vi "Lab2_FM.vi"() -> ()   [LabVIEW 2019]
uses:
  <vilib>/express/express analysis/Spectral/Block/exnSpectralBlock spectral measurements RMS poly.vi
  <vilib>/express/express analysis/Spectral/Block/exnSpectralBlock spectral measurements RMS DDT.vi
  <vilib>/express/express analysis/Spectral/XNode/ExpressSpectralMeasurementsBlockNode.xnode
panel:
  in  "stop":bool
  out "Time Domain":dynamicdata(graph)
  out "Freqency Domain":dynamicdata(graph)
  out "Carrier":dynamicdata(graph)
  out "Message":dynamicdata(graph)
  in  "Carrier Amplitude":dbl(slide) scale=0.0..10.0
  in  "Carrier Freqency":dbl(slide) scale=0.0..100000.0
  in  "Message Amplitude":dbl(slide) scale=0.0..10.0
  in  "Message Frequency":dbl(slide) scale=0.0..5000.0
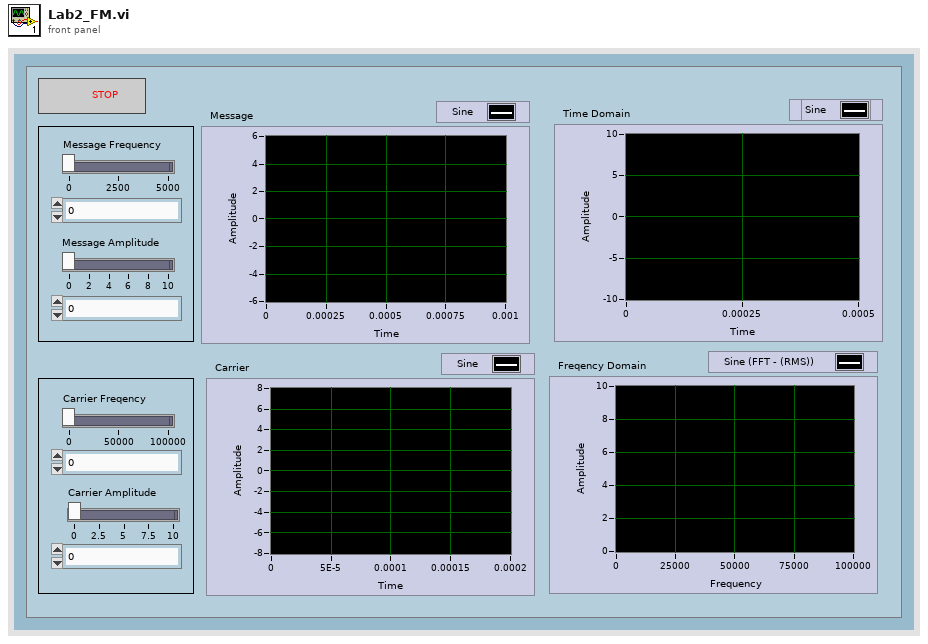
[diagram p1: front panel]
types:
  T1 = cluster{"averaging mode":u16, "weighting mode":u16, "number of averages":u32}
  T2 = cluster{"dB On (F)":bool, "unwrap phase (F)":bool, "convert to degree (F)":bool}
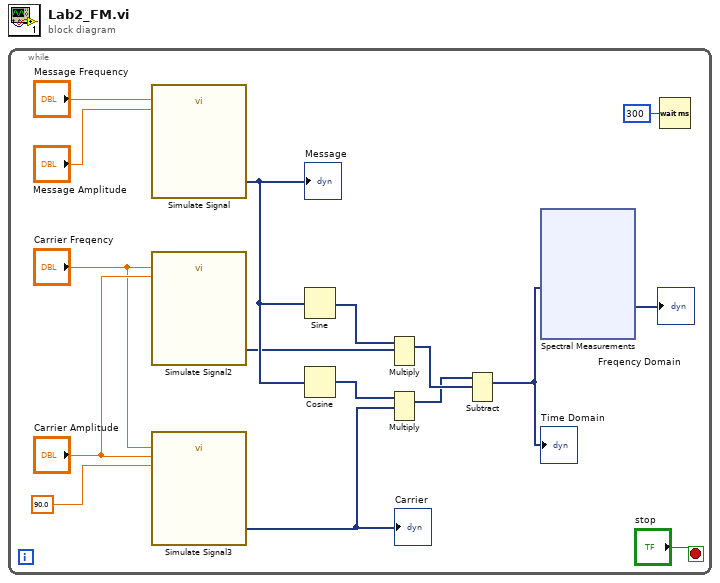
[diagram p0: block diagram]
diagram:
  n1 = while {
    stop <- "stop" stop-if-true
    n2 = call "Simulate Signal"("Frequency"="Message Frequency", "Amplitude"="Message Amplitude") -> ("Sine"=w9:dynamicdata)  [unwired: 12 in, 1 out]
    "Message" <- w9
    n3 = call "Simulate Signal2"("Frequency"="Carrier Freqency", "Amplitude"="Carrier Amplitude") -> ("Sine"=w8:dynamicdata)  [unwired: 12 in, 1 out]
    n4 = call "Simulate Signal3"("Frequency"="Carrier Freqency", "Amplitude"="Carrier Amplitude", "Phase"=90.0) -> ("Sine"=w12:dynamicdata)  [unwired: 11 in, 1 out]
    "Carrier" <- w12
    n5 = Sine(x=w9) -> (sin(x)=w10:dynamicdata)
    n6 = Cosine(x=w9) -> (cos(x)=w11:dynamicdata)
    n7 = Multiply(1:w8, 2:w10) -> (0:w5:dynamicdata)  [unwired: 1 in, 1 out]
    n8 = Multiply(1:w12, 2:w11) -> (0:w4:dynamicdata)  [unwired: 1 in, 1 out]
    n9 = Subtract(1:w5, 2:w4) -> (0:w3:dynamicdata)  [unwired: 1 in, 1 out]
    "Time Domain" <- w3
    n10 = xnode "Spectral Measurements"("Signals"=w3) -> ("FFT - (RMS)"=→"Freqency Domain":dynamicdata)  [unwired: 1 in, 2 out]
    n11 = Wait (ms)(milliseconds to wait=u32 300) -> ()  [unwired: 1 out]
  }
